vi "Read PL txt File.vi"(1 "Path":path) -> (0 "XY Graph":cluster{"all rows":dbl[], "all rows":dbl[]}(graph))   [LabVIEW 2011]
uses:
  <vilib>/Utility/file.llb/Read From Spreadsheet File (DBL).vi
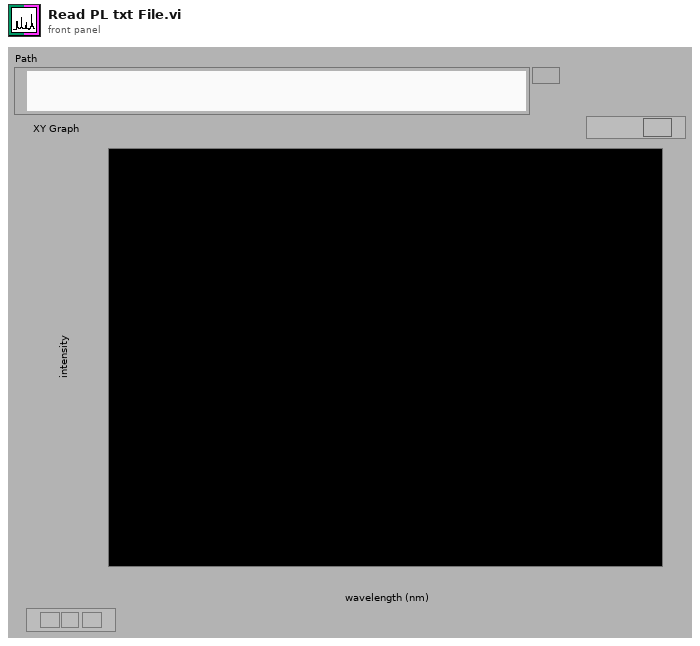
[diagram p1: front panel]
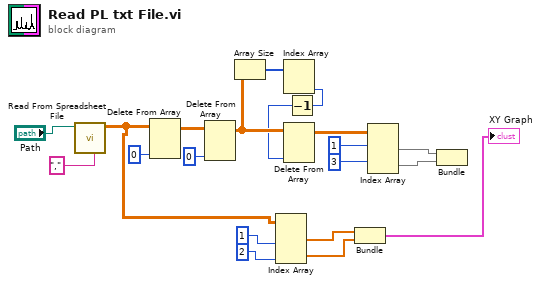
[diagram p0: block diagram]
diagram:
  n1 = call-poly <vilib>:"Read From Spreadsheet File.vi"("delimiter (\\t)"="," ("delimiter (\\t)"), "file path (dialog if empty)"="Path") -> ("all rows"=w6:dbl[][])  [unwired: 3 in, 6 out]
  n2 = Delete From Array(array=w6, index (col)=0 ("disabled index (col)")) -> (array with subset deleted=w18:dbl[][])  [unwired: 2 in, 1 out]
  n3 = Delete From Array(array=w18, index (col)=0 ("disabled index (col)")) -> (array with subset deleted=w11:dbl[][])  [unwired: 2 in, 1 out]
  n4 = Array Size(array=w11) -> (size(s)=w10:i32[])
  n5 = Index Array(array=w6, index (col) #1=1 ("index (row)"), index (col) #2=2 ("index (row)")) -> (element #1=w5:dbl[], element #2=w4:dbl[])  [unwired: 2 in]
  n6 = Index Array(array=w10) -> (element #2=w9:i32)  [unwired: 2 in, 1 out]
  n7 = Decrement(x=w9) -> (x-1=w8:i32)
  n8 = Delete From Array(array=w11, index (col)=w8) -> (array with subset deleted=w19:dbl[][])  [unwired: 2 in, 1 out]
  n9 = Bundle("all rows"=w5, "all rows"=w4) -> (→"XY Graph":cluster{"all rows":dbl[], "all rows":dbl[]})  [unwired: 1 out]
  n10 = Index Array(array=w19, index (row) #1=1 ("index (row)"), index (row) #2=3 ("index (row)")) -> (element #1=w15:dbl[], element #2=w14:dbl[])  [unwired: 2 in]
  n11 = Bundle("all rows"=w15, "all rows"=w14) -> ()  [unwired: 2 out]
